vi "Histogram PtByPt.vi"(6 "initialize":bool, 8 "sample length":i32=100, 10 "intervals":i32=10, 11 "x":dbl format="%0.2f") -> (0 "error":i32, 1 "X Values":dbl[](array[numeric]), 2 "Histogram: h(x)":i32[](array[numeric]), 3 "Histogram Graph":T1(graph))   [LabVIEW 2020, in "NI_PtbyPt.lvlib"]
doc: "Finds the discrete histogram of the set of input data points specified by <B>sample length</B>. The histogram is a frequency count of the number of times that a specified interval occurs in the set of input data points."
uses:
  <vilib>/ptbypt/NI_PtbyPt.lvlib
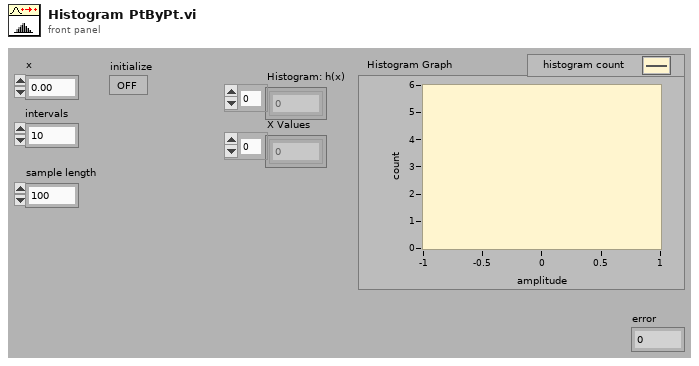
[diagram p1: front panel]
types:
  T1 = cluster{"X Values":dbl[], "Histogram: h(x)":i32[]}
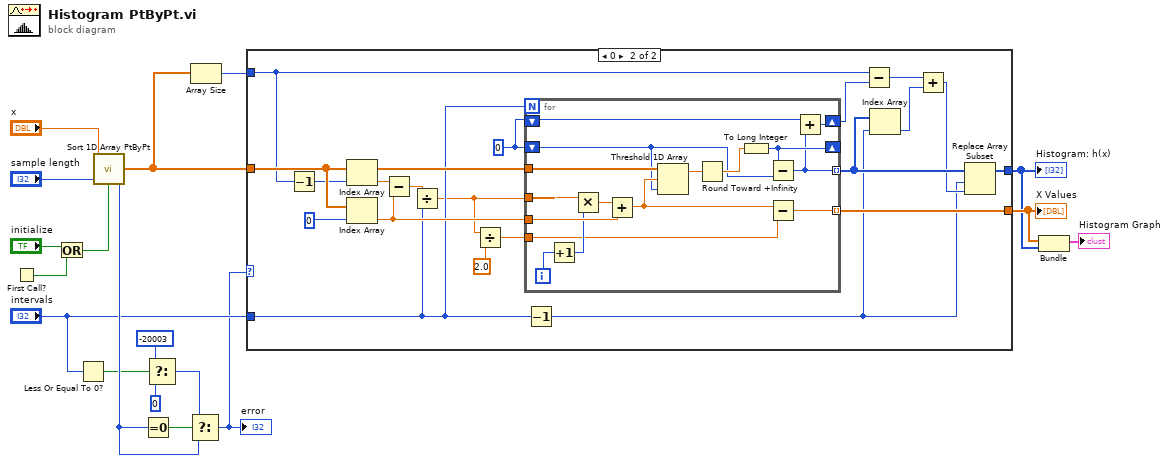
[diagram p0: block diagram]
diagram:
  n1 = First Call?() -> (First Call?: T/F=w14:bool)
  n2 = Or(x="initialize", y=w14) -> (x .or. y?=w16:bool)
  n3 = Less Or Equal To 0?(x="intervals") -> (x <= 0?=w11:bool)
  n4 = call <vilib>:"Sort 1D Array PtByPt.vi"("initialize"=w16, "sample length"="sample length", "input data point"="x") -> ("error"=w17:i32, "sorted array"=w2:dbl[])  [unwired: 1 in]
  n5 = Equal To 0?(x=w17) -> (x = 0?=w10:bool)
  n6 = Select(t=-20003, s=w11, f=0) -> (s? t:f=w9:i32)
  n7 = Select(t=w9, s=w10, f=w17) -> (s? t:f=w7:i32)
  "error" <- w7
  n8 = Array Size(array=w2) -> (size(s)=w1:i32)
  n9 = case shown="0" w7 {
    tunnel: [_ w34] -> w6
    tunnel: [_ w33] -> w5
    tunnel: w2 -> [_ w32]
    tunnel: "intervals" -> [_ w31]
    tunnel: w1 -> [_ w23]
    frame -1, Default {
    }
    frame 0 {
      w30 = 0
      n10 = Decrement(x=w23) -> (x-1=w27:i32)
      n11 = Index Array(array=w32, index=w27) -> (element=w37:dbl)
      n12 = Index Array(array=w32, index=0 ("Index")) -> (element=w35:dbl)
      n13 = Subtract(x=w37, y=w35) -> (x-y=w36:dbl)
      n14 = Divide(x=w36, y=w31) -> (x/y=w25:dbl)
      n15 = Divide(x=w25, y=2.0) -> (x/y=w24:dbl)
      n16 = for {
        N: w31 -> [_]
        tunnel: w25 -> [w46]
        tunnel: w35 -> [w48]
        tunnel: w32 -> [w53]
        tunnel: [w41] -> w28 mode=indexing
        tunnel: [w47] -> w34 mode=indexing
        shift-right: [w49] -> _
        shift-left: w30 -> [w39]
        shift-right: [w42] -> w29
        shift-left: w30 -> [w43]
        tunnel: w24 -> [w40]
        i -> [w45]
        n17 = Increment(x=w45) -> (x+1=w44:i32)
        n18 = Multiply(x=w46, y=w44) -> (x*y=w54:dbl)
        n19 = Add(x=w54, y=w48) -> (x+y=w52:dbl)
        n20 = Threshold 1D Array(1:w39, 2:w52, 3:w53) -> (0:w51:dbl)
        n21 = Round Toward +Infinity(x=w51) -> (ceil(x): smallest int >= x=w50:dbl)
        n22 = To Long Integer(number=w50) -> (32bit integer=w49:i32)
        n23 = Subtract(x=w49, y=w39) -> (x-y=w41:i32)
        n24 = Subtract(x=w52, y=w40) -> (x-y=w47:dbl)
        n25 = Add(x=w43, y=w41) -> (x+y=w42:i32)
      }
      n26 = Decrement(x=w31) -> (x-1=w19:i32)
      n27 = Subtract(x=w23, y=w29) -> (x-y=w21:i32)
      n28 = Index Array(array=w28, index=w19) -> (element=w22:i32)
      n29 = Add(x=w21, y=w22) -> (x+y=w20:i32)
      n30 = Replace Array Subset(array=w28, new element=w20, index=w19) -> (w33:i32[])
    }
  }
  "Histogram: h(x)" <- w5
  "X Values" <- w6
  n31 = Bundle(w6, w5) -> (→"Histogram Graph":cluster{dbl[], i32[]})  [unwired: 1 in]
